vi "Launch Topic.vi"(7 "Include Initial Value? (F)":bool, 9 "Type":variant, 10 "Datum Name":string, 11 "Mediator in":refnum<class "Mediator.lvclass">) -> (0 "error out":errorcluster, 2 "New Topic Enqueuer":refnum<class "Message Enqueuer.lvclass">, 3 "Mediator out":refnum<class "Mediator.lvclass">)   [LabVIEW 2017, in "MyMediator.lvlib副本.lvlib" / "Mediator.lvclass"]
uses:
  Mediator.lvclass
  C:/Program Files (x86)/National Instruments/LabVIEW 2017/vi.lib/ActorFramework/Actor/Actor.lvclass
  C:/Program Files (x86)/National Instruments/LabVIEW 2017/vi.lib/Composed/GPM Packages/mva-framework/Source/Framework/IMediator/IMediator/IMediator.lvclass
  <vilib>/ActorFramework/Message Enqueuer/Message Enqueuer.lvclass
  <vilib>/Composed/GPM Packages/mva-framework/Source/Framework/IMediator/IMediator/IMediator.lvclass/IMediator.ctl
  <vilib>/Composed/GPM Packages/mva-framework/Source/Framework/SubscriptionPolicy/BasicSubscription/BasicSubscription.lvclass/BasicSubscription.ctl
  Topic/Topic.lvclass/Topic.ctl
  Mediator.lvclass/Mediator.ctl
  TopicLookupTable/TopicLookupTable.lvclass/TopicLookupTable.ctl
  <vilib>/Composed/GPM Packages/transport/Source/Concrete/ActorMessageTransport/ActorMessageTransport.lvclass/ActorMessageTransport.ctl
  Topic Messages/Add Topic Subscriber Msg/Add Topic Subscriber Msg.lvclass/Add Topic Subscriber Msg.ctl
  <vilib>/ActorFramework/Message Enqueuer/Message Enqueuer.lvclass/Message Enqueuer.ctl
  Topic/Read Topic Info.vi
  <vilib>/ActorFramework/Message Enqueuer/Equals Not A Refnum.vi
  <vilib>/ActorFramework/Message Enqueuer/Enqueue.vi
  <vilib>/ActorFramework/Actor/Read Self Enqueuer.vi
  <vilib>/ActorFramework/Message Enqueuer/Init from Existing Queue.vi
  <vilib>/Composed/GPM Packages/mva-framework/Source/Framework/SubscriptionPolicy/BasicSubscription/BasicSubscription.lvclass
  C:/Program Files (x86)/National Instruments/LabVIEW 2017/vi.lib/Composed/GPM Packages/mva-framework/Source/Framework/IMediator/ISubscriptionPolicy/ISubscriptionPolicy.lvclass
  Topic/Topic.lvclass
  <vilib>/Composed/GPM Packages/transport/Source/Concrete/ActorMessageTransport/ActorMessageTransport.lvclass
  C:/Program Files (x86)/National Instruments/LabVIEW 2017/vi.lib/Composed/GPM Packages/transport/Source/ITransport/ITransport.lvclass
  Topic Messages/Add Topic Subscriber Msg/Add Topic Subscriber Msg.lvclass
  C:/Program Files (x86)/National Instruments/LabVIEW 2017/vi.lib/ActorFramework/Message/Message.lvclass
  <vilib>/ActorFramework/Message Priority Queue/Priority Enqueue.vi
  <vilib>/Utility/error.llb/Error Cluster From Error Code.vi
  <vilib>/Composed/GPM Packages/variant/Source/Format Type String.vi
  <vilib>/Composed/GPM Packages/transport/Source/Concrete/ActorMessageTransport/Notification Msg/Notification Msg.lvclass
  <vilib>/ActorFramework/Actor/Actor.lvclass
  TopicLookupTable/TopicLookupTable.lvclass
  <vilib>/Composed/GPM Packages/mva-framework/Source/Framework/IMediator/ISubscriptionPolicy/ISubscriptionPolicy.lvclass
  <vilib>/Composed/GPM Packages/mva-framework/Source/Framework/IMediator/IMediator/IMediator.lvclass
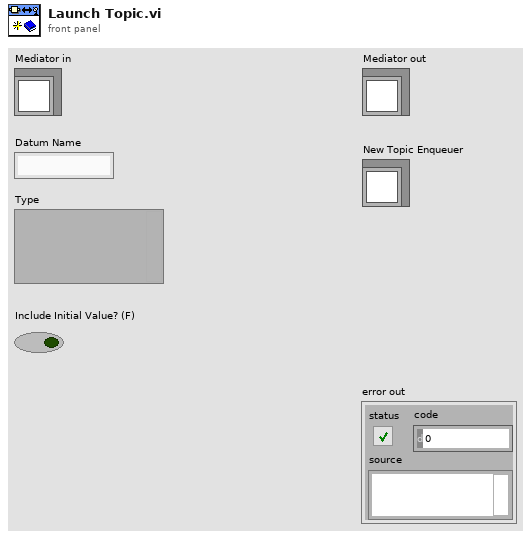
[diagram p1: front panel]
types:
  T1 = typedef "IMediator.lvlib/ISubscriptionPolicy.lvclass/ISubscriptionPolicy Reference.ctl" = refnum<data-value>
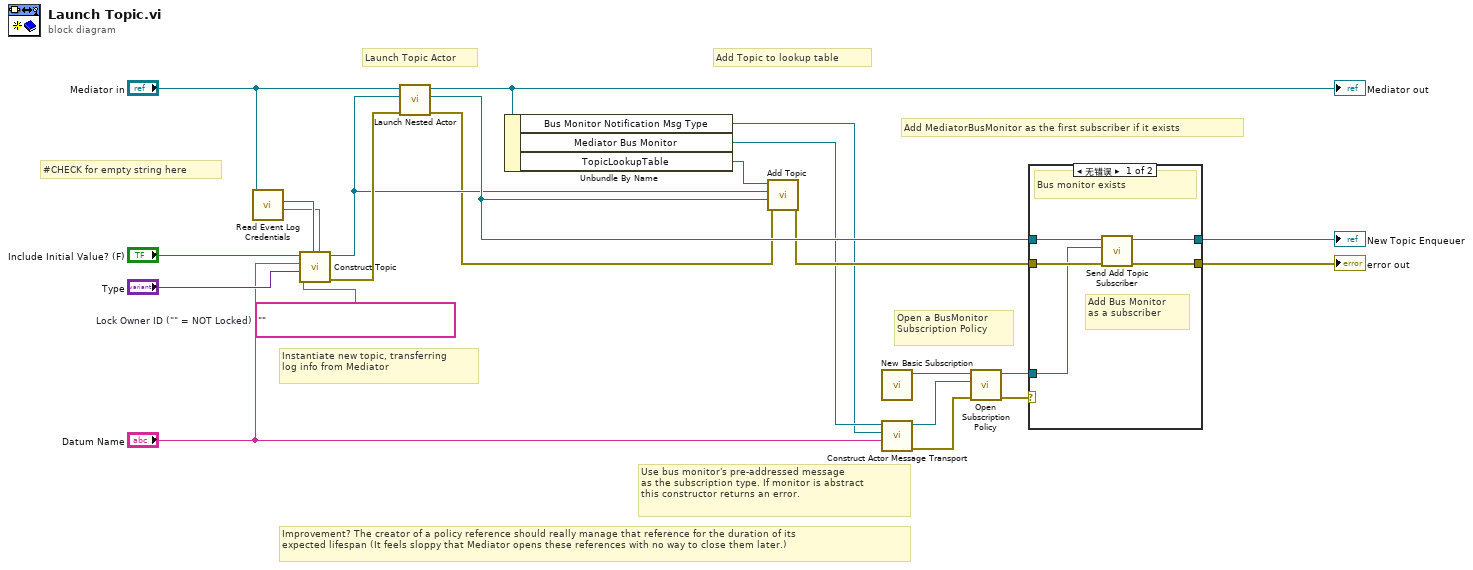
[diagram p0: block diagram]
diagram:
  w11 = ""  # Lock Owner ID ("" = NOT Locked)
  # "#CHECK for empty string here"
  # "Open a BusMonitor\nSubscription Policy"
  # "Use bus monitor's pre-addressed message\nas the subscription type. If monitor is abstract\nthis constructor returns an error."
  # "Improvement? The creator of a policy reference should really manage that reference for the duration of its\nexpected lifespan (It feels sloppy that Mediator opens these references with no way to close them later.)"
  # "Add MediatorBusMonitor as the first subscriber if it exists"
  # "Launch Topic Actor"
  # "Add Topic to lookup table"
  # "Instantiate new topic, transferring\nlog info from Mediator"
  n1 = call <vilib>:"Read Event Log Credentials.vi"("IMediator in"="Mediator in") -> ("Framework Instance Alias"=w4:string, "Event Log Instance"=w5:refnum<class "LoggerReference.lvclass">)  [unwired: 9 in]
  n2 = call "Construct Topic.vi"("Framework Instance Alias"=w4, "Event Log Instance"=w5, "Lock Owner ID (\"\" = NOT Locked)"=w11, "New Topic Data"="Type", "Name"="Datum Name", "Use Type Input As Initial Value?"="Include Initial Value? (F)") -> ("error out"=w20:errorcluster, "Topic out"=w19:refnum<class "Topic.lvclass">)  [unwired: 4 in]
  n3 = call <vilib>:"Launch Nested Actor.vi"("error in (no error)"=w20, "Nested Actor"=w19, "Caller Actor in"="Mediator in") -> ("error out"=w1:errorcluster, "Nested Actor's Enqueuer"=w21:refnum<class "Message Enqueuer.lvclass">, "Caller Actor out"=w15:refnum<class "Mediator.lvclass">)  [unwired: 6 in]
  "Mediator out" <- w15
  n4 = Unbundle By Name(w15) -> ("Bus Monitor Notification Msg Type"=w7:refnum<class "Notification Msg.lvclass">, "Mediator Bus Monitor"=w13:refnum<class "Message Enqueuer.lvclass">, "TopicLookupTable"=w18:refnum<data-value>)
  n5 = call "Add Topic.vi"("error in (no error)"=w1, "Topic Enqueuer"=w21, "Topic Object"=w19, "TopicLookupTable"=w18) -> ("error out"=w17:errorcluster)  [unwired: 5 in, 2 out]
  n6 = call <vilib>:"New Basic Subscription.vi"() -> ("BasicSubscription Out"=w9:refnum<class "BasicSubscription.lvclass">)  [unwired: 11 in]
  n7 = call <vilib>:"Construct Actor Message Transport.vi"("Datum Name"="Datum Name", "Notification Msg"=w7, "Message Enqueuer in"=w13) -> ("error out"=w3:errorcluster, "ActorMessageTransport"=w10:refnum<class "ActorMessageTransport.lvclass">)  [unwired: 7 in]
  n8 = call <vilib>:"Open Subscription Policy.vi"("error in (no error)"=w3, "Transport"=w10, "SubscriptionPolicy"=w9) -> ("error out"=w2:errorcluster, "Subscription Policy"=w8:T1)  [unwired: 7 in]
  n9 = case shown="无错误" w2 {
    tunnel: [w28 w30] -> w22
    tunnel: w21 -> [w27 w30]
    tunnel: w17 -> [w26 w29]
    tunnel: [w25 w29] -> w16
    tunnel: w8 -> [w24 _]
    frame No Error {
      # "Add Bus Monitor\nas a subscriber"
      # "Bus monitor exists"
      n10 = call "Send Add Topic Subscriber.vi"("error in (no error)"=w26, "Subscription Policy"=w24, "Message Enqueuer"=w27) -> ("error out"=w25:errorcluster, "Message Enqueuer out"=w28:refnum<class "Message Enqueuer.lvclass">)  [unwired: 7 in]
    }
    frame Error {
      # "No bus monitor"
    }
  }
  "error out" <- w16
  "New Topic Enqueuer" <- w22
